vi "DAQmx_Analogue_Measurement.vi"(5 "Input ranges":dbl[](array[numeric]), 6 "Sampling rate":dbl format="%#_13g", 7 "Output ranges":dbl[](array[numeric]), 8 "error in":errorcluster, 9 "Input channels":cluster{string, "physical channels":tag}[](array[cluster]), 10 "Output channels":cluster{string, "physical channels":tag}[](array[cluster])=[{"ao0", "physical channels"="Dev1/ao0"}, {"ao1", "physical channels"="Dev1/ao1"}], 11 "Outputs":waveform(dbl)[](array[waveform])) -> (0 "error out":errorcluster, 2 "Measured data":waveform(dbl)[](array[waveform]))   [LabVIEW 2016]
uses:
  <vilib>/DAQmx/write.llb/DAQmx Write (Analog 1D Wfm NChan NSamp).vi
  <vilib>/DAQmx/read.llb/DAQmx Read (Analog 1D Wfm NChan NSamp).vi
  <vilib>/DAQmx/write.llb/DAQmx Write (Analog 1D DBL NChan 1Samp).vi
  <vilib>/DAQmx/create/channels.llb/DAQmx Create Channel (AO-Voltage-Basic).vi
  <vilib>/DAQmx/configure/timing.llb/DAQmx Timing (Sample Clock).vi
  <vilib>/DAQmx/miscellaneous.llb/DAQmx Fill In Error Info.vi
  <vilib>/DAQmx/create/channels.llb/DAQmx Create Channel (AI-Voltage-Basic).vi
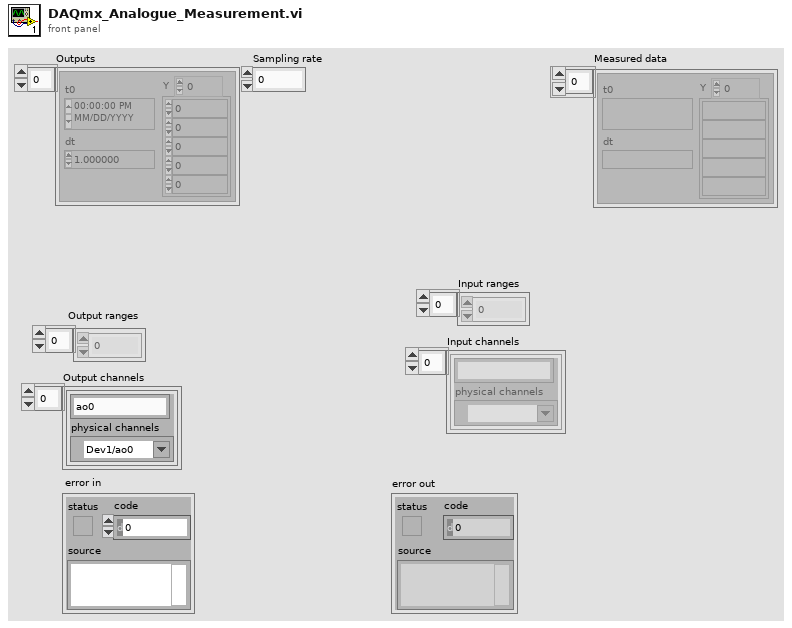
[diagram p1: front panel]
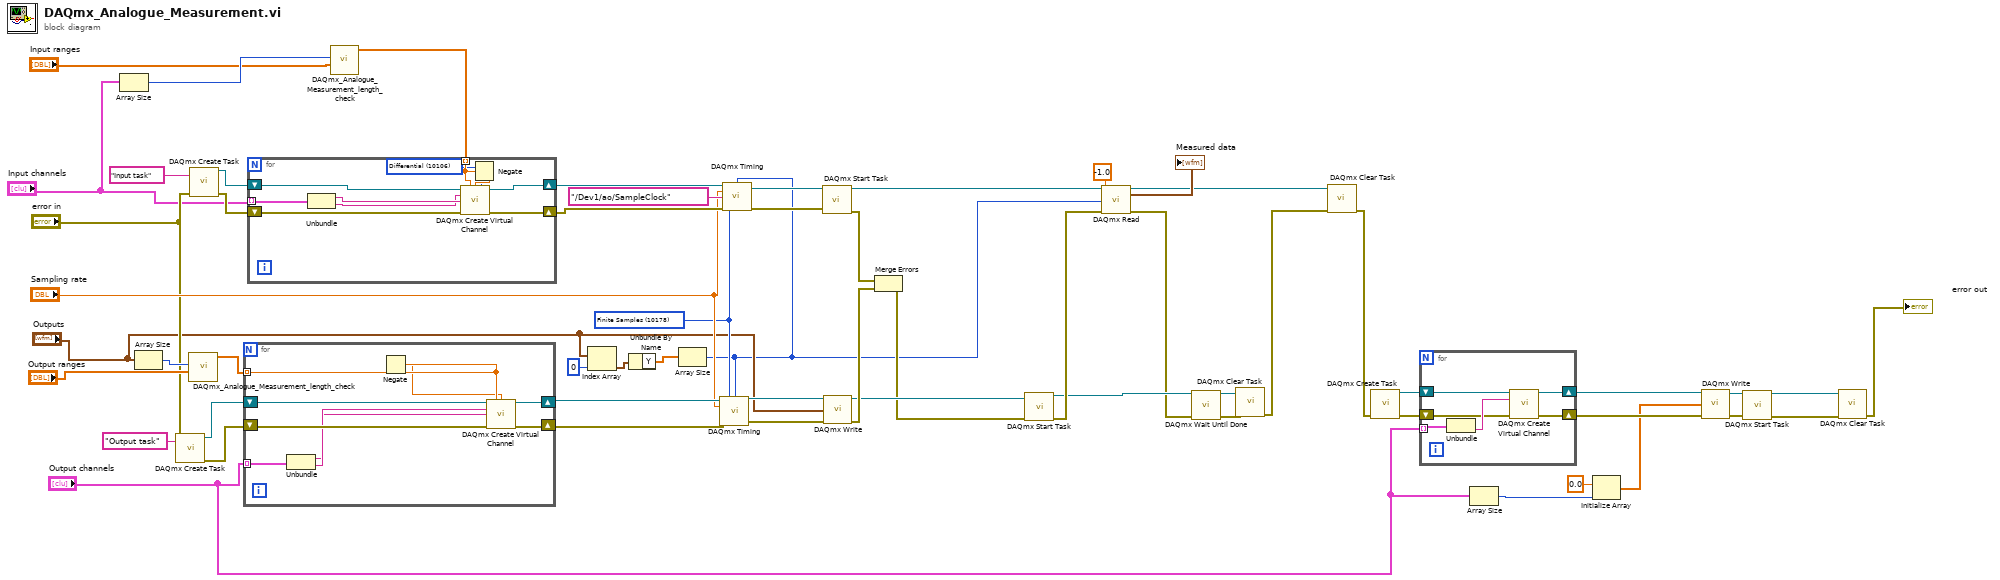
[diagram p0: block diagram]
diagram:
  w40 = 10178 items=["Finite Samples"=10178, "Continuous Samples"=10123, "Hardware Timed Single Point"=12522] ("sample mode")
  n1 = Array Size(array="Input channels") -> (size(s)=w55:i32)
  n2 = Array Size(array="Outputs") -> (size(s)=w51:i32)
  n3 = call <vilib>:"DAQmx Create Task.vi"("new task name"="Output task", "error in"="error in") -> ("task out"=w48:refnum<k21>, "error out"=w47:errorcluster)  [unwired: 12 in]
  n4 = call "DAQmx_Analogue_Measurement_length_check.vi"("Input ranges in"="Output ranges", "Requested length"=w51) -> ("Input ranges out"=w49:dbl[])  [unwired: 9 in]
  n5 = call <vilib>:"DAQmx Create Task.vi"("new task name"="Input task", "error in"="error in") -> ("task out"=w57:refnum<k21>, "error out"=w54:errorcluster)  [unwired: 12 in]
  n6 = for {
    tunnel: w49 -> [w67] mode=indexing
    shift-right: [w64] -> w43
    shift-left: w48 -> [w65]
    shift-right: [w62] -> w42
    shift-left: w47 -> [w63]
    tunnel: "Output channels" -> [w61] mode=indexing
    n7 = Unbundle(w61) -> (w59:string, "physical channels"=w60:tag)
    n8 = Negate(x=w67) -> (-x=w66:dbl)
    n9 = call-poly <vilib>:"DAQmx Create Virtual Channel.vi"("task in"=w65, "maximum value"=w67, "minimum value"=w66, "physical channels"=w60, "name to assign"=w59, "error in"=w63) -> ("task out"=w64:refnum<k21>, "error out"=w62:errorcluster)  [unwired: 8 in]
  }
  n10 = call "DAQmx_Analogue_Measurement_length_check.vi"("Input ranges in"="Input ranges", "Requested length"=w55) -> ("Input ranges out"=w56:dbl[])  [unwired: 9 in]
  n11 = for {
    tunnel: "Input channels" -> [w70] mode=indexing
    shift-right: [w76] -> w46
    shift-left: w57 -> [w77]
    tunnel: w56 -> [w74] mode=indexing
    shift-right: [w73] -> w45
    shift-left: w54 -> [w72]
    w71 = 10106 items=["Default"=-1, "RSE"=10083, "NRSE"=10078, "Differential"=10106, "Pseudodifferential"=12529] ("input terminal configuration")
    n12 = Unbundle(w70) -> (w69:string, "physical channels"=w68:tag)
    n13 = Negate(x=w74) -> (-x=w75:dbl)
    n14 = call-poly <vilib>:"DAQmx Create Virtual Channel.vi"("task in"=w77, "maximum value"=w74, "minimum value"=w75, "input terminal configuration"=w71, "physical channels"=w68, "name to assign"=w69, "error in"=w72) -> ("task out"=w76:refnum<k21>, "error out"=w73:errorcluster)  [unwired: 7 in]
  }
  n15 = Index Array(array="Outputs", index=0) -> (element=w23:waveform(dbl))
  n16 = Unbundle By Name(w23) -> ("Y"=w22:dbl[])
  n17 = Array Size(array=w22) -> (size(s)=w19:i32)
  n18 = call-poly <vilib>:"DAQmx Timing.vi"("task/channels in"=w43, "sample mode"=w40, "samples per channel"=w19, "rate"="Sampling rate", "error in"=w42) -> ("task out"=w39:refnum<k21>, "error out"=w38:errorcluster)  [unwired: 9 in]
  n19 = call-poly <vilib>:"DAQmx Timing.vi"("task/channels in"=w46, "sample mode"=w40, "samples per channel"=w19, "rate"="Sampling rate", "source"=tag "/Dev1/ao/SampleClock", "error in"=w45) -> ("task out"=w37:refnum<k21>, "error out"=w36:errorcluster)  [unwired: 8 in]
  n20 = call <vilib>:"DAQmx Start Task.vi"("task/channels in"=w37, "error in"=w36) -> ("task out"=w31:refnum<k21>, "error out"=w34:errorcluster)  [unwired: 12 in]
  n21 = call-poly <vilib>:"DAQmx Write.vi"("task/channels in"=w39, "data"="Outputs", "error in"=w38) -> ("task out"=w32:refnum<k21>, "error out"=w35:errorcluster)  [unwired: 10 in, 1 out]
  n22 = Merge Errors(w34, w35) -> (w26:errorcluster)
  n23 = call <vilib>:"DAQmx Start Task.vi"("task/channels in"=w32, "error in"=w26) -> ("task out"=w29:refnum<k21>, "error out"=w33:errorcluster)  [unwired: 12 in]
  n24 = call-poly <vilib>:"DAQmx Read.vi"("task/channels in"=w31, "number of samples per channel"=w19, "timeout"=-1.0, "error in"=w33) -> ("task out"=w17:refnum<k21>, "data"=→"Measured data":waveform(dbl)[], "error out"=w16:errorcluster)  [unwired: 9 in]
  n25 = call <vilib>:"DAQmx Wait Until Done.vi"("task/channels in"=w29, "error in"=w16) -> ("task out"=w25:refnum<k21>, "error out"=w24:errorcluster)  [unwired: 12 in]
  n26 = call <vilib>:"DAQmx Clear Task.vi"("task in"=w25, "error in"=w24) -> ("error out"=w18:errorcluster)  [unwired: 13 in]
  n27 = call <vilib>:"DAQmx Clear Task.vi"("task in"=w17, "error in"=w18) -> ("error out"=w14:errorcluster)  [unwired: 13 in]
  n28 = call <vilib>:"DAQmx Create Task.vi"("error in"=w14) -> ("task out"=w13:refnum<k21>, "error out"=w12:errorcluster)  [unwired: 13 in]
  n29 = for {
    tunnel: "Output channels" -> [w81] mode=indexing
    shift-right: [w82] -> w11
    shift-left: w13 -> [w83]
    shift-right: [w78] -> w10
    shift-left: w12 -> [w79]
    n30 = Unbundle(w81) -> ("physical channels"=w80:tag)  [unwired: 1 out]
    n31 = call-poly <vilib>:"DAQmx Create Virtual Channel.vi"("task in"=w83, "physical channels"=w80, "error in"=w79) -> ("task out"=w82:refnum<k21>, "error out"=w78:errorcluster)  [unwired: 11 in]
  }
  n32 = Array Size(array="Output channels") -> (size(s)=w8:i32)
  n33 = Initialize Array(0.0 ("element"), w8) -> (w6:dbl[])
  n34 = call-poly <vilib>:"DAQmx Write.vi"("task/channels in"=w11, "data"=w6, "error in"=w10) -> ("task out"=w5:refnum<k21>, "error out"=w4:errorcluster)  [unwired: 10 in, 1 out]
  n35 = call <vilib>:"DAQmx Start Task.vi"("task/channels in"=w5, "error in"=w4) -> ("task out"=w2:refnum<k21>, "error out"=w1:errorcluster)  [unwired: 12 in]
  n36 = call <vilib>:"DAQmx Clear Task.vi"("task in"=w2, "error in"=w1) -> ("error out"=→"error out":errorcluster)  [unwired: 13 in]
